vi "Untitled 3.vi"() -> ()   [LabVIEW 2012]
uses:
  <vilib>/addons/database/NI_Database_API.lvlib
  <vilib>/addons/database/Connection.llb/DB Tools Open Connec (Path).vi
  <vilib>/addons/database/Connection.llb/Conn Execute.vi
  <vilib>/addons/database/Recordset.llb/Rec Fetch Recordset Data (R).vi
  <vilib>/addons/database/Recordset.llb/Rec Destroy - Connection.vi
  <vilib>/addons/database/_DB Variant To Data/Database Variant To Data.xnode
panel:
  out "appended array":string[](array[string])
  out "data":string
  out "trimmed string":string
  out "data 2":string
  out "error out":errorcluster
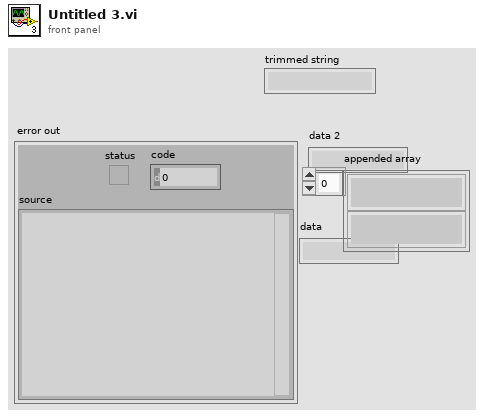
[diagram p1: front panel]
types:
  T1 = typedef "NI_Database_API.lvlib/Conn ObjectReference.ctl" = refnum<k1>
  T2 = typedef "NI_Database_API.lvlib/Rec ObjectReference.ctl" = refnum<k1>
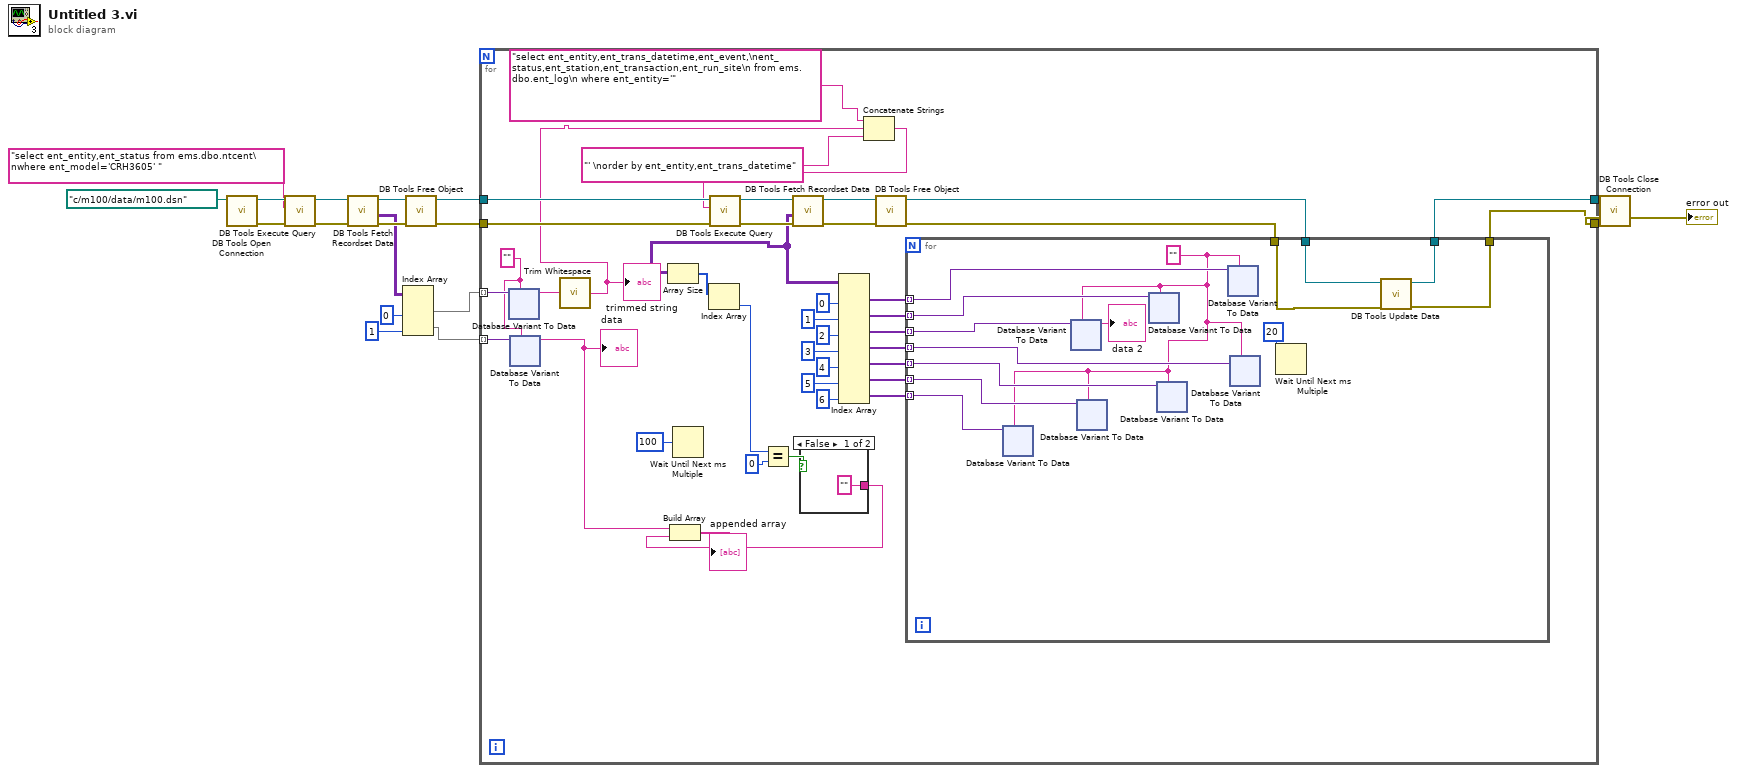
[diagram p0: block diagram]
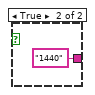
[diagram p2: hidden frame]
diagram:
  n1 = call-poly <vilib>:"DB Tools Open Connection.vi"("connection information"=path "c:/m100/data/m100.dsn") -> ("error out"=w10:errorcluster, "connection reference"=w17:T1)  [unwired: 7 in]
  n2 = call-poly <vilib>:"DB Tools Execute Query.vi"("error in (no error)"=w10, "SQL query"="select ent_entity,ent_status from ems.dbo.ntcent\nwhere ent_model='CRH3605' ", "connection reference"=w17) -> ("error out"=w11:errorcluster, "recordset reference"=w16:T2)  [unwired: 5 in]
  n3 = call-poly <vilib>:"DB Tools Fetch Recordset Data.vi"("error in (no error)"=w11, "recordset reference"=w16) -> ("error out"=w12:errorcluster, "recordset data"=w8:variant[][], "recordset reference out"=w15:T2)  [unwired: 3 in]
  n4 = Index Array(array=w8, index (col) #1=0 ("disabled index (col)"), index (col) #2=1 ("index (col)")) -> (element #1=w6:variant[], element #2=w1:variant[])  [unwired: 2 in]
  n5 = call-poly <vilib>:"DB Tools Free Object.vi"("error in (no error)"=w12, "recordset reference"=w15) -> ("error out"=w13:errorcluster, "connection reference"=w14:T1)  [unwired: 8 in]
  n6 = for {
    tunnel: w14 -> [w42]
    tunnel: w13 -> [w41]
    tunnel: w6 -> [w39] mode=indexing
    tunnel: [w20] -> w5
    tunnel: [w19] -> w4
    tunnel: w1 -> [w33] mode=indexing
    w32 = ""
    n7 = xnode "Database Variant To Data"("database variant"=w39, "type"=w32) -> ("data"=w36:string)  [unwired: 1 in, 1 out]
    n8 = xnode "Database Variant To Data"("database variant"=w33, "type"=w32) -> ("data"=w26:string)  [unwired: 1 in, 1 out]
    "data" <- w26
    n9 = call <vilib>:"Trim Whitespace.vi"("string"=w36) -> ("trimmed string"=w34:string)  [unwired: 1 in]
    "trimmed string" <- w34
    n10 = Wait Until Next ms Multiple(millisecond multiple=u32 100) -> ()  [unwired: 1 out]
    n11 = Concatenate Strings("select ent_entity,ent_trans_datetime,ent_event,\nent_status,ent_station,ent_transaction,ent_run_site\n from ems.dbo.ent_log\n where ent_entity='" ("SQL query"), w34, "' \norder by ent_entity,ent_trans_datetime" ("string")) -> (w37:string)
    n12 = call-poly <vilib>:"DB Tools Execute Query.vi"("error in (no error)"=w41, "SQL query"=w37, "connection reference"=w42) -> ("error out"=w57:errorcluster, "recordset reference"=w59:T2)  [unwired: 5 in]
    n13 = call-poly <vilib>:"DB Tools Fetch Recordset Data.vi"("error in (no error)"=w57, "recordset reference"=w59) -> ("error out"=w56:errorcluster, "recordset data"=w31:variant[][], "recordset reference out"=w58:T2)  [unwired: 3 in]
    n14 = Array Size(array=w31) -> (size(s)=w30:i32[])
    n15 = Index Array(array=w30) -> (element=w29:i32)  [unwired: 1 in]
    n16 = Equal?(x=w29, y=0) -> (x = y?=w27:bool)
    n17 = case shown="False" w27 {
      tunnel: ["" "1440"] -> w25
      frame False {
      }
      frame True {
      }
    }
    n18 = Build Array(w26, w25) -> (→"appended array":string[])
    n19 = Index Array(array=w31, index (col) #1=0 ("disabled index (col)"), index (col) #2=1 ("index (col)"), index (col) #3=2 ("index (col)"), index (col) #4=3 ("index (col)"), index (col) #5=4 ("index (col)"), index (col) #6=5 ("index (col)"), index (col) #7=6 ("index (col)")) -> (element #1=w48:variant[], element #2=w47:variant[], element #3=w46:variant[], element #4=w40:variant[], element #5=w45:variant[], element #6=w44:variant[], element #7=w43:variant[])  [unwired: 7 in]
    n20 = call-poly <vilib>:"DB Tools Free Object.vi"("error in (no error)"=w56, "recordset reference"=w58) -> ("error out"=w21:errorcluster, "connection reference"=w22:T1)  [unwired: 8 in]
    n21 = for {
      tunnel: w48 -> [w139] mode=indexing
      tunnel: w47 -> [w138] mode=indexing
      tunnel: w46 -> [w137] mode=indexing
      tunnel: w45 -> [w135] mode=indexing
      tunnel: w40 -> [w136] mode=indexing
      tunnel: w44 -> [w134] mode=indexing
      tunnel: w43 -> [w133] mode=indexing
      tunnel: w22 -> [w129]
      tunnel: w21 -> [w128]
      tunnel: [w127] -> w20
      tunnel: [w126] -> w19
      w132 = ""
      n22 = xnode "Database Variant To Data"("database variant"=w133, "type"=w132) -> ()  [unwired: 1 in, 2 out]
      n23 = xnode "Database Variant To Data"("database variant"=w137, "type"=w132) -> ("data"=→"data 2":string)  [unwired: 1 in, 1 out]
      n24 = xnode "Database Variant To Data"("database variant"=w134, "type"=w132) -> ()  [unwired: 1 in, 2 out]
      n25 = xnode "Database Variant To Data"("database variant"=w138, "type"=w132) -> ()  [unwired: 1 in, 2 out]
      n26 = xnode "Database Variant To Data"("database variant"=w135, "type"=w132) -> ()  [unwired: 1 in, 2 out]
      n27 = xnode "Database Variant To Data"("database variant"=w139, "type"=w132) -> ()  [unwired: 1 in, 2 out]
      n28 = xnode "Database Variant To Data"("database variant"=w136, "type"=w132) -> ()  [unwired: 1 in, 2 out]
      n29 = Wait Until Next ms Multiple(millisecond multiple=u32 20) -> ()  [unwired: 1 out]
      n30 = call <vilib>:"DB Tools Update Data.vi"("error in (no error)"=w128, "connection reference"=w129) -> ("error out"=w126:errorcluster, "connection reference out"=w127:T1)  [unwired: 8 in]
    }
  }
  n31 = call <vilib>:"DB Tools Close Connection.vi"("error in (no error)"=w4, "connection reference"=w5) -> ("error out"=→"error out":errorcluster)  [unwired: 5 in]
